vi "duplicate.vi"(8 "error in (no error)":errorcluster, 11 "TestCase in":refnum<class "TestCase.Pointer.lvclass">) -> (0 "error out":errorcluster, 3 "TestCase out":refnum<class "TestCase.Pointer.lvclass">)   [LabVIEW 2016, in "TestCase.Pointer.lvclass"]
uses:
  TestCase.Pointer.lvclass
  TestCase.Pointer.lvclass/TestCase.Pointer.ctl
  Source/Classes/Pointer/Memory.Pointer.lvclass/Memory.Pointer.ctl
  Source/Classes/Internal/Memory.Pointer.Internal.New.vi
  Source/Classes/Pointer/Memory.Pointer.Get Size.vi
  Source/Classes/Pointer/Memory.Pointer.Copy All.vi
  Source/Classes/Pointer/Memory.Pointer.Copy All.Safe.vi
  Source/Classes/Pointer/Memory.Pointer.Copy.Safe.vi
  Source/Classes/Pointer/Memory.Pointer.Copy.Unsafe.vi
  Source/Classes/Pointer/Memory.Pointer.Parameter Check.Subset.vi
  Source/Classes/Pointer/Memory.Pointer.Parameter Check.Null Pointer.vi
  Source/Classes/Pointer/Memory.Pointer.Get Address.vi
  Source/Classes/Pointer/Memory.Pointer.Errors.vi
  Source/Classes/Pointer/Memory.Pointer.Errors.Out of Bounds.vi
  Source/Classes/Pointer/Memory.Pointer.Errors.Null Pointer.vi
  Source/Submodules/SEH/Source/VIs/Static Error Handling.Source Buffer.Write.String.vi
  Source/Classes/Pointer/Memory.Pointer.Errors.Write Pointer Size.vi
  Source/Classes/Pointer/Memory.Pointer.Errors.Create Error.vi
  Source/Submodules/SEH/Source/VIs/Static Error Handling.Source Buffer.Write.Numeric.Scalar.Base10.vi
  Source/Submodules/SEH/Source/VIs/Static Error Handling.Source Buffer.Write.Numeric.Scalar.Base10 (U64).vi
  Source/Submodules/SEH/Source/VIs/Static Error Handling.Error Cluster Constant.vi
  Source/Submodules/SEH/Source/VIs/Static Error Handling.Error Cluster Constant (256B).vi
  Source/Submodules/SEH/Source/VIs/Static Error Handling.Parameters.Status.Set.vi
  Source/Submodules/SEH/Source/VIs/Static Error Handling.Parameters.Code.Set.vi
  Source/Submodules/SEH/Source/VIs/Static Error Handling.Parameters.VI Source.Set.vi
  Source/Constants/Memory.Constants.vi
  Source/Constants/Memory.Constants.Library Name.vi
  Source/Classes/Pointer/Memory.Pointer.Errors.Get Info.vi
  Source/Classes/Internal/Memory.Pointer.Internal.lvclass
  C:/Git/Sourcetree/LabVIEW-Memory/Source/Classes/Pointer/Memory.Pointer.lvclass
  Source/Classes/Internal/Memory.Pointer.Internal.Allocate.vi
  <vilib>/addons/_JKI Toolkits/VI Tester/TestCase.llb/TestCase.lvclass
  Source/Classes/Pointer/Memory.Pointer.lvclass
  C:/Program Files (x86)/National Instruments/LabVIEW 2016/vi.lib/addons/_JKI Toolkits/VI Tester/TestCase.llb/TestCase.lvclass
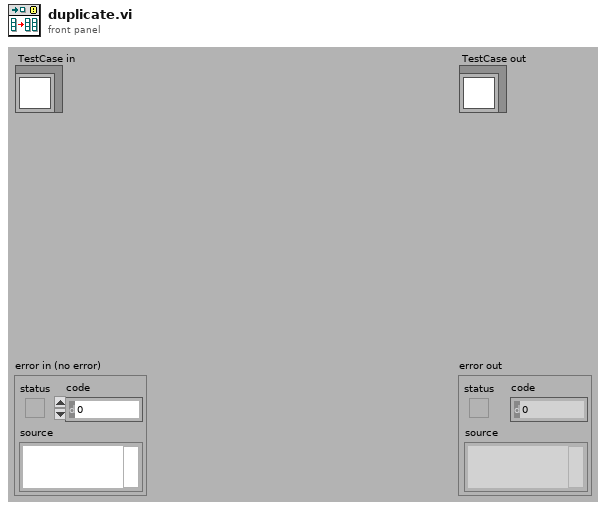
[diagram p1: front panel]
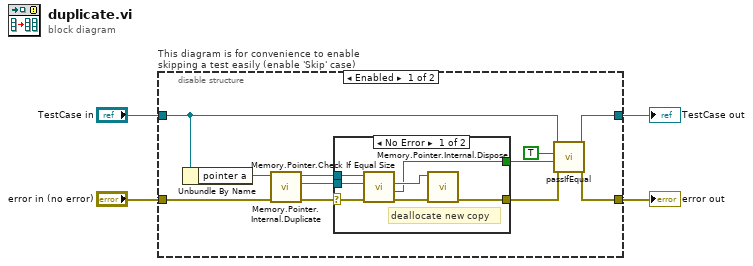
[diagram p0: block diagram]
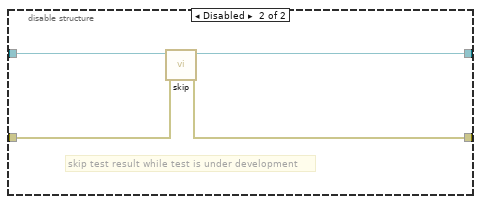
[diagram p3: hidden frame]
diagram:
  n1 = disable-structure "This diagram is for convenience to enable skipping a test easily (enable 'Skip' case)" shown="Enabled" {
    disable-tunnel: "TestCase in" -> [w13 w27]
    disable-tunnel: [w15 w25] -> w1
    disable-tunnel: [w14 w26] -> w3
    disable-tunnel: "error in (no error)" -> [w11 w24]
    frame Enabled {
      n2 = Unbundle By Name(w13) -> ("pointer a"=w12:refnum<class "Memory.Pointer.Internal.lvclass">)
      n3 = call "Memory.Pointer.Internal.Duplicate.vi"("error in (no error)"=w11, "pointer in"=w12) -> ("error out"=w10:errorcluster, "new pointer"=w7:refnum<class "Memory.Pointer.Internal.lvclass">, "pointer out"=w8:refnum<class "Memory.Pointer.Internal.lvclass">)  [unwired: 7 in]
      n4 = case shown="No Error" w10 {
        selector: w10 -> [w20 w23]
        tunnel: w8 -> [w22 _]
        tunnel: w7 -> [w21 _]
        tunnel: [w17 w23] -> w6
        tunnel: [w16 _] -> w5
        frame No Error {
          # "deallocate new copy"
          n5 = call "Memory.Pointer.Check If Equal Size.vi"("error in (no error)"=w20, "pointer b in"=w21, "pointer a in"=w22) -> ("error out"=w19:errorcluster, "equal size?"=w16:bool, "pointer b out"=w18:refnum<class "Memory.Pointer.Internal.lvclass">)  [unwired: 5 in, 1 out]
          n6 = call "Memory.Pointer.Internal.Dispose.vi"("error in (no error)"=w19, "pointer"=w18) -> ("error out"=w17:errorcluster)  [unwired: 9 in]
        }
        frame Error {
        }
      }
      n7 = call-dynamic "passIfEqual.vi"("error in (no error)"=w6, "y"=w5, "x"=TRUE, "TestCase in"=w13) -> ("error out"=w14:errorcluster, "TestCase out"=w15:refnum<class "TestCase.Pointer.lvclass">)  [unwired: 6 in]
    }
    frame Disabled {
      # "skip test result while test is under development"
      n8 = call <vilib>:"skip.vi"("error in (no error)"=w24, "TestCase in"=w27) -> ("error out"=w26:errorcluster, "TestCase out"=w25:refnum<class "TestCase.Pointer.lvclass">)  [unwired: 8 in]
    }
  }
  "error out" <- w3
  "TestCase out" <- w1
